vi "LVClass_Image dtor.vi"(0 "Image in":refnum<class "Image.lvclass">, 11 "error in (no error)":errorcluster) -> (4 "Image out":refnum<class "Image.lvclass">, 15 "error out":errorcluster)   [LabVIEW 2020, in "Image.lvclass"]
doc: "Image destructor.\n\n--------------------------------------------------------------------------------\n\n<B>ImageIn </B> : Image object.\n<B>ImageOut </B> : Image object.\n<B>ErrorIn </B> : Error\n<B>ErrorOut </B> : Error\n\n--------------------------------------------------------------------------------"
uses:
  Image.lvclass
  Image.lvclass/Image.ctl
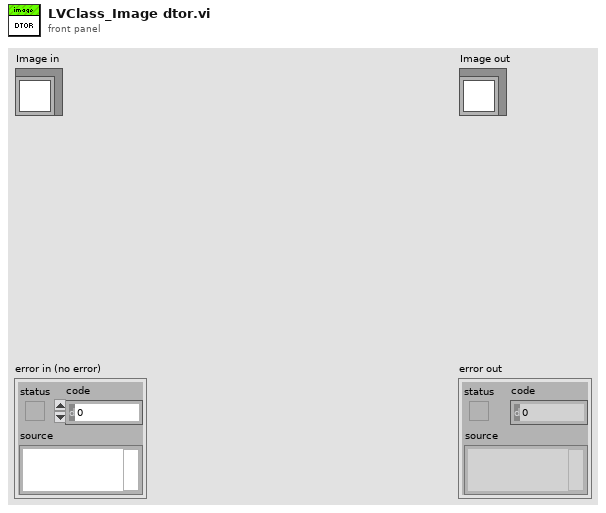
[diagram p1: front panel]
types:
  T1 = typedef "Handle creation.ctl" = enum16{"By ctor", "By write function"}
  T2 = typedef "ClassID.ctl" = i64
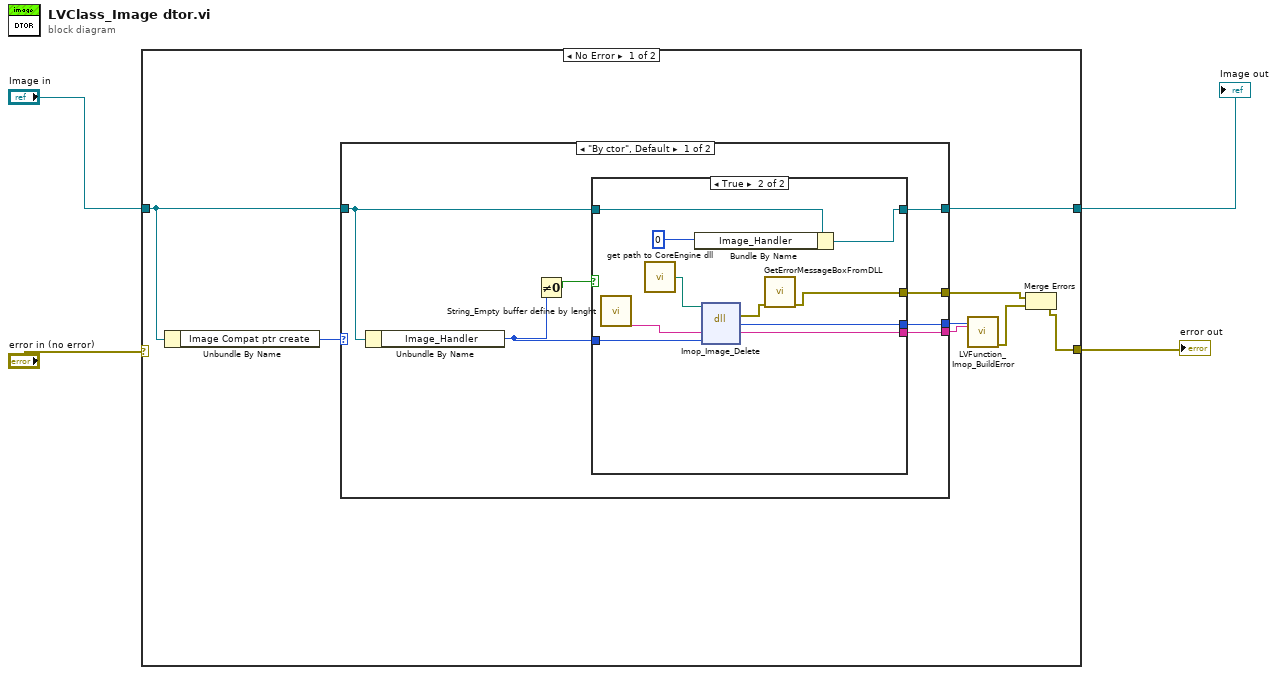
[diagram p0: block diagram]
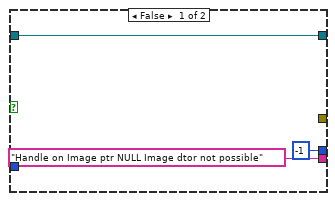
[diagram p2: hidden frame]
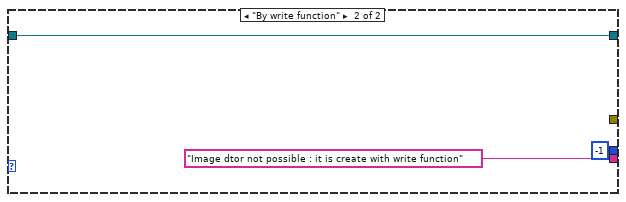
[diagram p3: hidden frame]
diagram:
  n1 = case shown="No Error" "error in (no error)" {
    selector: "error in (no error)" -> [_ w36]
    tunnel: "Image in" -> [w9 w37]
    tunnel: [w10 w37] -> w3
    tunnel: [w5 w36] -> w1
    frame No Error {
      n2 = Unbundle By Name(w9) -> ("Image Compat ptr create"=w8:T1)
      n3 = case shown="\"By ctor\", Default" w8 {
        tunnel: [w19 w35] -> w10
        tunnel: [w18 -1] -> w12
        tunnel: [w17 "Image dtor not possible : it is create with write function" ("message")] -> w11
        tunnel: w9 -> [w14 w35]
        tunnel: [w13 _] -> w7
        frame "By ctor", Default {
          n4 = Unbundle By Name(w14) -> ("Image_Handler"=w15:T2)
          n5 = Not Equal To 0?(x=w15) -> (x != 0?=w16:bool)
          n6 = case shown="True" w16 {
            tunnel: w14 -> [w22 w31]
            tunnel: [w22 w30] -> w19
            tunnel: [-1 w28] -> w18
            tunnel: ["Handle on Image ptr NULL Image dtor not possible" ("message") w27] -> w17
            tunnel: w15 -> [_ w26]
            tunnel: [_ w23] -> w13
            frame False {
            }
            frame True {
              n7 = call "String_Empty buffer define by lenght.vi"() -> ("Empty buffer"=w32:string)  [unwired: 1 in]
              n8 = call "get path to CoreEngine dll.vi"() -> ("path to wavekit library"=w25:path)  [unwired: 14 in, 1 out]
              n9 = Bundle By Name(cluster=w31, "Image_Handler"=0 ("Image Compat ptr")) -> (w30:refnum<class "Image.lvclass">)
              n10 = dll-call lib="D:/soft/HASO_v3/SVN_trunk/ImOpCoreEngine4_LV2011/DLLs/c_interface_vc100.dll" fn="Imop_Image_Delete"(path in=w25, "message"=w32, "objet"=w26) -> (error out=w24:errorcluster, "return type"=w28:i32, "message"=w27:string)  [unwired: 3 in, 1 out]
              n11 = call "GetErrorMessageBoxFromDLL.vi"("error IN"=w24) -> ("error OUT"=w23:errorcluster)  [unwired: 10 in]
            }
          }
        }
        frame "By write function" {
        }
      }
      n12 = call "LVFunction_Imop_BuildError.vi"("code"=w12, "String to Prepend to source (\"\")"=w11) -> ("error out"=w6:errorcluster)  [unwired: 13 in]
      n13 = Merge Errors(w7, w6) -> (w5:errorcluster)
    }
    frame Error {
    }
  }
  "error out" <- w1
  "Image out" <- w3
